vi "APS get first axis Id.vi"(8 "error in (no error)":errorcluster caption="错误输入（无错误）", 9 "TotalAxisNum":i32, 10 "StartAxisID":i32, 11 "Board_ID":i32) -> (0 "error out":errorcluster caption="错误输出", 1 "TotalAxisNum out":i32, 2 "StartAxisID out":i32, 3 "function return":i32)   [LabVIEW 2011, in "APS168.lvlib"]
doc: "I32 FNTYPE APS_get_first_axisId( I32 Board_ID, I32 *StartAxisID, I32 *TotalAxisNum );"
uses:
  APS168.lvlib
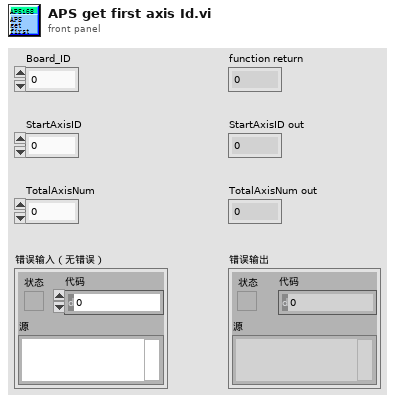
[diagram p1: front panel]
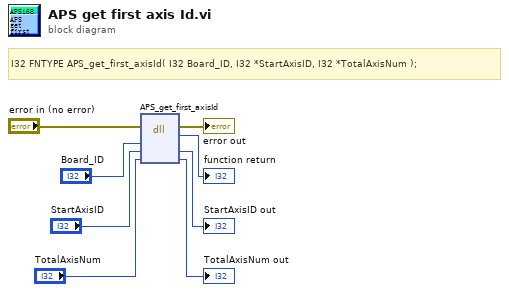
[diagram p0: block diagram]
diagram:
  # "I32 FNTYPE APS_get_first_axisId( I32 Board_ID, I32 *StartAxisID, I32 *TotalAxisNum );"
  n1 = dll-call lib="PTH1Labs E软件ADLINK 204CAPS_1_7_1_LIB line 连续运动204APS168.*" fn="APS_get_first_axisId"(error in="error in (no error)", "Board_ID"="Board_ID", "StartAxisID"="StartAxisID", "TotalAxisNum"="TotalAxisNum") -> (error out=→"error out":errorcluster, →"function return":i32, "StartAxisID"=→"StartAxisID out":i32, "TotalAxisNum"=→"TotalAxisNum out":i32)  [unwired: 3 in, 1 out]
